vi "NF90.vi"() -> ()   [LabVIEW 2010]
doc: "Illustrates the simplest form of TCP data acquisition using a TCP data server.\n\n\nCreated by Monroe Weber-Shirk\nCornell University\nmw24@cornell.edu\nJanuary 2000"
uses:
  NF90 move.ctl
  Axis.ctl
  NF90 commands.ctl
panel:
  out "position (xyz)":dbl[](array[numeric])
  in  "Go to Start":bool
  in  "Go Home":bool
  in  "Done":bool
  in  "Find Home":bool
  in  "axis":T1=enum."Z"
  in  "Acceleration":u8=1 min=1 max=50 step=1
  in  "Speed":sgl=1.0 min=0 max=3 format="%.3f"
  in  "Target position":sgl min=-1048575 max=1048575 step=1 format="%.2f"
  in  "move":T2={"axis"=enum."Z", "Increment"=0.0, "Speed"=1.0, "Acceleration"=1} {"Speed" min=0 format="%.3f"; "Acceleration" min=1 max=50 step=1; "Increment" format="%.3f"}
  in  "Home offset from limit switch":sgl min=-1048575 max=1048575 step=1 format="%.2f"
  in  "port number":refnum<visa-resource-name>="COM1"
  # "cm"
  # "cm"
  # "cm"
  # "cm"
  # "cm/s"
  # "cm/s^2"
  # "cm"
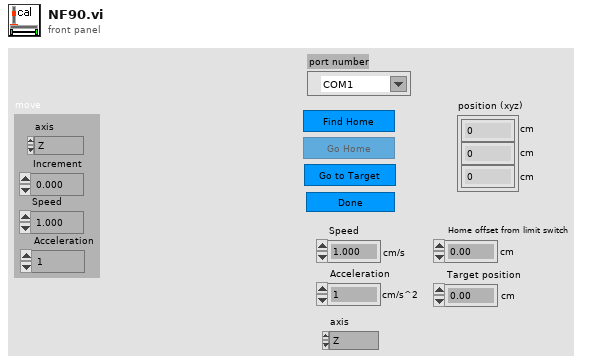
[diagram p1: front panel]
types:
  T1 = typedef "Axis.ctl" = enum16{"X", "Y", "Z"}
  T2 = typedef "NF90 move.ctl" = cluster{"axis":T1, "Increment":sgl, "Speed":sgl, "Acceleration":u8}
  T3 = typedef "NF90 commands.ctl" = enum16{"Index", "Speed", "Acceleration", "Backlash", "Quit", "Run", "Null indexes", "Verify status", "Clear program", "Computer Control", "Go", "Put Controller on Hold", "Position"}
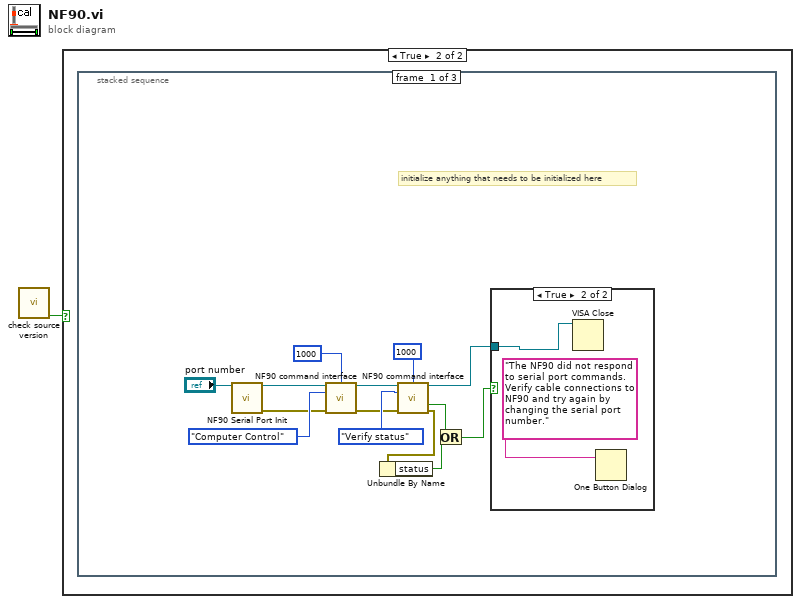
[diagram p0: block diagram]
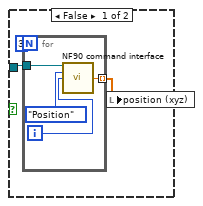
[diagram p3: hidden frame]
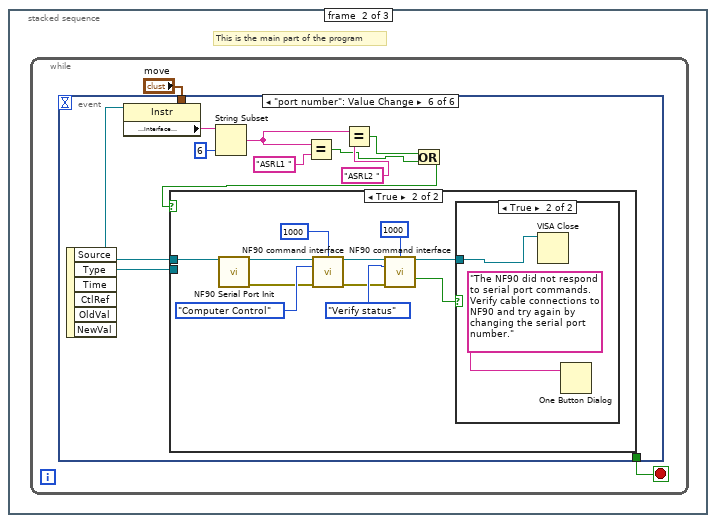
[diagram p4: hidden frame]
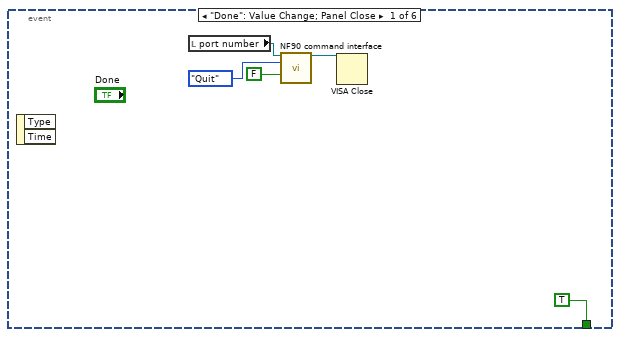
[diagram p5: hidden frame]
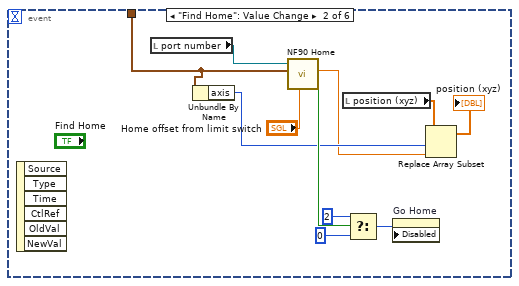
[diagram p6: hidden frame]
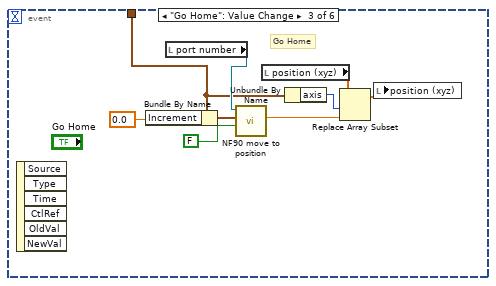
[diagram p7: hidden frame]
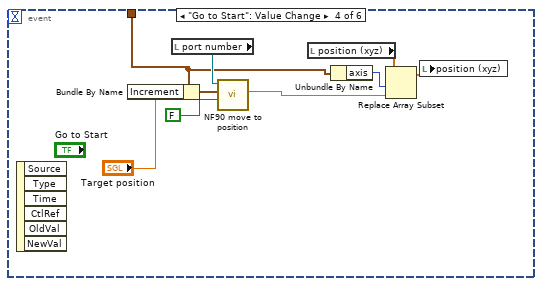
[diagram p8: hidden frame]
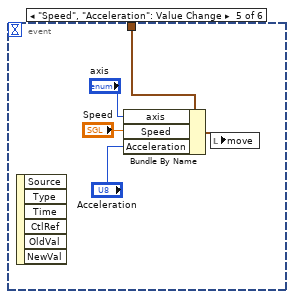
[diagram p9: hidden frame]
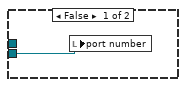
[diagram p10: hidden frame]
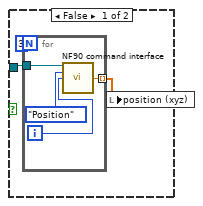
[diagram p11: hidden frame]
diagram:
  n1 = call "check source version.vi"() -> ("continue running?"=w1:bool)  [unwired: 2 in, 3 out]
  n2 = case shown="True" w1 {
    frame False {
    }
    frame True {
      n3 = stacked-sequence {
        frame #0 {
          # "initialize anything that needs to be initialized here"
          n4 = call "NF90 Serial Port Init.vi"("port number"="port number") -> ("port number"=w15:refnum<visa-resource-name>, "error out"=w9:errorcluster)  [unwired: 13 in]
          n5 = call "NF90 command interface.vi"("port number in"=w15, "time out (ms)"=u32 1000, "commands"=NF90_commands."Computer Control", "Error In"=w9) -> ("port number out"=w12:refnum<visa-resource-name>, "Error Out"=w8:errorcluster)  [unwired: 7 in, 3 out]
          n6 = call "NF90 command interface.vi"("port number in"=w12, "time out (ms)"=u32 1000, "commands"=NF90_commands."Verify status", "Error In"=w8) -> ("port number out"=w2:refnum<visa-resource-name>, "timed out"=w6:bool, "Error Out"=w5:errorcluster)  [unwired: 7 in, 2 out]
          n7 = Unbundle By Name(w5) -> ("status"=w7:bool)
          n8 = Or(x=w6, y=w7) -> (x .or. y?=w3:bool)
          n9 = case shown="True" w3 {
            tunnel: w2 -> [w18 w23]
            frame False {
              n10 = for {
                N: 3 -> [_]
                tunnel: w18 -> [w21]
                tunnel: [w19] -> w17 mode=indexing
                i -> [w20]
                n11 = call "NF90 command interface.vi"("port number in"=w21, "commands"=NF90_commands."Position", "axis"=w20) -> ("Position"=w19:sgl)  [unwired: 8 in, 4 out]
              }
              n12 = local write "position (xyz)"(w17) -> ()
            }
            frame True {
              n13 = VISA Close(VISA resource name=w23) -> ()  [unwired: 1 in, 1 out]
              n14 = One Button Dialog(message="The NF90 did not respond to serial port commands. Verify cable connections to NF90 and try again by changing the serial port number.") -> ()  [unwired: 1 in, 1 out]
            }
          }
        }
        frame #1 {
          # "This is the main part of the program"
          n15 = while {
            stop <- w25 stop-if-true
            n16 = event shown="[5] \"port number\": Value Change" {
              selector: _ -> [_ _ _ _ _ _]
              dyn-events: _ -> [_ _ _ _ _ _]
              timeout: _ -> [_ _ _ _ _ _]
              tunnel: "move" -> [_ w34 w46 w52 w61 _]
              tunnel: [TRUE ("quit") _ _ _ _ _] -> w25
              event "Done": Value Change; Panel Close {
                n17 = event-data() -> ()  [unwired: 1 in, 2 out]
                n18 = local read "port number"() -> (w28:refnum<visa-resource-name>)
                n19 = call "NF90 command interface.vi"("port number in"=w28, "commands"=NF90_commands."Quit", "enable?"=FALSE) -> ("port number out"=w31:refnum<visa-resource-name>)  [unwired: 8 in, 4 out]
                n20 = VISA Close(VISA resource name=w31) -> ()  [unwired: 1 in, 1 out]
              }
              event "Find Home": Value Change {
                n21 = event-data() -> ()  [unwired: 1 in, 6 out]
                n22 = local read "port number"() -> (w37:refnum<visa-resource-name>)
                n23 = Unbundle By Name(w34) -> ("axis"=w33:T1)
                n24 = call "NF90 Home.vi"("Index offset from switch"="Home offset from limit switch", "move"=w34, "port number in"=w37) -> ("killed"=w39:bool, "position"=w32:dbl)  [unwired: 4 in, 2 out]
                n25 = local read "position (xyz)"() -> (w36:dbl[])
                n26 = Select(t=2, s=w39, f=0) -> (s? t:f=w41:i32)
                n27 = property on="Go Home" class="Bool"("Disabled"=w41) -> ()  [unwired: 2 in, 2 out]
                n28 = Replace Array Subset(array=w36, new element=w32, index=w33) -> (→"position (xyz)":dbl[])
              }
              event "Go Home": Value Change {
                # "Go Home"
                n29 = event-data() -> ()  [unwired: 1 in, 6 out]
                n30 = Bundle By Name(cluster=w46, "Increment"=sgl 0.0 ("Bundle Element")) -> (w49:T2)
                n31 = local read "port number"() -> (w48:refnum<visa-resource-name>)
                n32 = call "NF90 move to position.vi"("move type (abs = False)"=FALSE ("move type (abs = true)"), "move"=w49, "port number in"=w48) -> ("Position out"=w45:sgl)  [unwired: 4 in, 3 out]
                n33 = local read "position (xyz)"() -> (w47:dbl[])
                n34 = Unbundle By Name(w46) -> ("axis"=w44:T1)
                n35 = Replace Array Subset(array=w47, new element=w45, index=w44) -> (w43:dbl[])
                n36 = local write "position (xyz)"(w43) -> ()
              }
              event "Go to Start": Value Change {
                n37 = event-data() -> ()  [unwired: 1 in, 6 out]
                n38 = Bundle By Name(cluster=w52, "Increment"="Target position") -> (w58:T2)
                n39 = local read "port number"() -> (w57:refnum<visa-resource-name>)
                n40 = call "NF90 move to position.vi"("move type (abs = False)"=FALSE ("move type (abs = true)"), "move"=w58, "port number in"=w57) -> ("Position out"=w53:sgl)  [unwired: 4 in, 3 out]
                n41 = local read "position (xyz)"() -> (w56:dbl[])
                n42 = Unbundle By Name(w52) -> ("axis"=w55:T1)
                n43 = Replace Array Subset(array=w56, new element=w53, index=w55) -> (w54:dbl[])
                n44 = local write "position (xyz)"(w54) -> ()
              }
              event "Speed", "Acceleration": Value Change {
                n45 = event-data() -> ()  [unwired: 1 in, 6 out]
                n46 = Bundle By Name(cluster=w61, "axis"="axis", "Speed"="Speed", "Acceleration"="Acceleration") -> (w64:T2)
                n47 = local write "move"(w64) -> ()
              }
              event "port number": Value Change {
                n48 = event-data() -> ("OldVal"=w66:refnum<visa-resource-name>, "NewVal"=w67:refnum<visa-resource-name>)  [unwired: 1 in, 4 out]
                n49 = property class="Instr"(reference=w67) -> ("Interface Information:Interface Description"=w70:string)  [unwired: 1 in, 2 out]
                n50 = String Subset(string=w70, length (rest)=6 ("length (rest)")) -> (substring=w69:string)  [unwired: 1 in]
                n51 = Equal?(x=w69, y="ASRL1 ") -> (x = y?=w72:bool)
                n52 = Equal?(x=w69, y="ASRL2 ") -> (x = y?=w73:bool)
                n53 = Or(x=w73, y=w72) -> (x .or. y?=w71:bool)
                n54 = case shown="True" w71 {
                  tunnel: w67 -> [_ w77]
                  tunnel: w66 -> [w76 _]
                  frame False {
                    n55 = local write "port number"(w76) -> ()
                  }
                  frame True {
                    n56 = call "NF90 Serial Port Init.vi"("port number"=w77) -> ("port number"=w87:refnum<visa-resource-name>, "error out"=w79:errorcluster)  [unwired: 13 in]
                    n57 = call "NF90 command interface.vi"("port number in"=w87, "time out (ms)"=u32 1000, "commands"=NF90_commands."Computer Control", "Error In"=w79) -> ("port number out"=w84:refnum<visa-resource-name>, "Error Out"=w78:errorcluster)  [unwired: 7 in, 3 out]
                    n58 = call "NF90 command interface.vi"("port number in"=w84, "time out (ms)"=u32 1000, "commands"=NF90_commands."Verify status", "Error In"=w78) -> ("port number out"=w83:refnum<visa-resource-name>, "timed out"=w80:bool)  [unwired: 7 in, 3 out]
                    n59 = case shown="True" w80 {
                      tunnel: w83 -> [w90 w95]
                      frame False {
                        n60 = for {
                          N: 3 -> [_]
                          tunnel: w90 -> [w93]
                          tunnel: [w91] -> w89 mode=indexing
                          i -> [w92]
                          n61 = call "NF90 command interface.vi"("port number in"=w93, "commands"=NF90_commands."Position", "axis"=w92) -> ("Position"=w91:sgl)  [unwired: 8 in, 4 out]
                        }
                        n62 = local write "position (xyz)"(w89) -> ()
                      }
                      frame True {
                        n63 = VISA Close(VISA resource name=w95) -> ()  [unwired: 1 in, 1 out]
                        n64 = One Button Dialog(message="The NF90 did not respond to serial port commands. Verify cable connections to NF90 and try again by changing the serial port number.") -> ()  [unwired: 1 in, 1 out]
                      }
                    }
                  }
                }
              }
            }
          }
        }
        frame #2 {
        }
      }
    }
  }
